vi "2-1.vi"() -> ()   [LabVIEW 2012]
doc: "© Copyright M. Ferrari 1999"
panel:
  out "Waveform Chart":dbl(graph)
  out "data out":dbl(knob) scale=0.0..10.0 scale format="%#_4g"
  out "low limit":dbl(knob) scale=10.0..100.0 scale format="%#_4g"
  out "hight limit":dbl(knob) scale=10.0..100.0 scale format="%#_4g"
  out "data in":dbl format="%.2f"
  in  "control":bool
  # "Se control = ON, bisogna verificare che il valore sia compreso nei limiti\n                     trasferendo il valore di ingresso diviso per il range ( hight limit-low limit)\n                     in uscita; se il valore  \"data in\"  non rientra nei limiti, oppure\nse control = OFF, non viene effettuato nessun controllo e il valore di ingresso passa\n                    direttamente in uscita"
  # "far apparire la scritta ON ,\no la scritta OFF, a seconda\ndei casi, su sfondo bianco"
  # "sostituire con un indicatore \ndi tipo ' meter' con indicatore digitale"
  # "sostituire con due controlli \ndi tipo ' knob' con indicatore digitale"
  # "Eliminare dal pannello tutte le indicazioni in arancio"
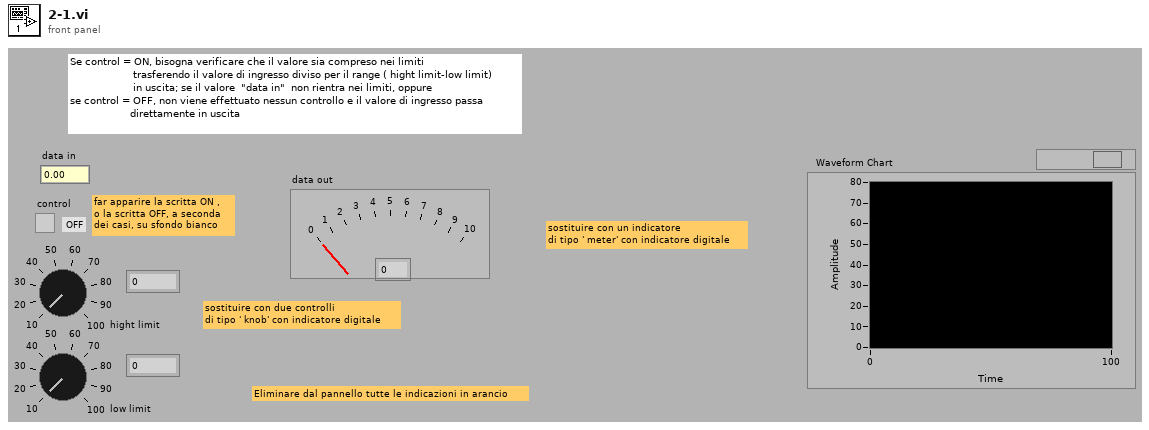
[diagram p1: front panel]
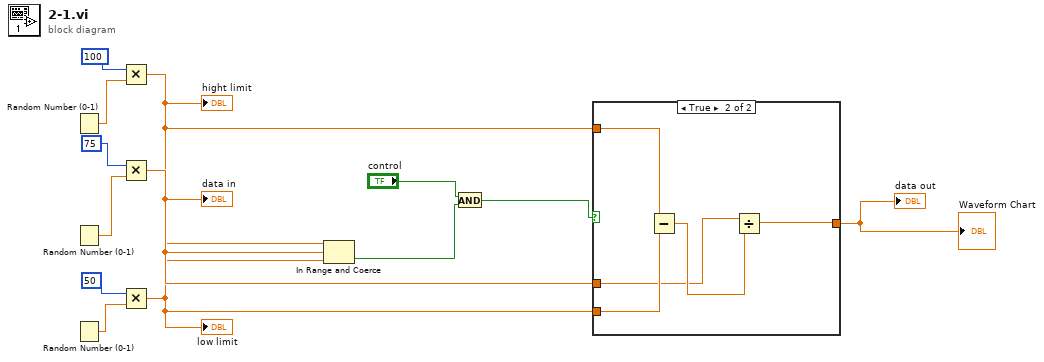
[diagram p0: block diagram]
diagram:
  n1 = Random Number (0-1)() -> (number: 0 to 1=w6:dbl)
  n2 = Random Number (0-1)() -> (number: 0 to 1=w10:dbl)
  n3 = Random Number (0-1)() -> (number: 0 to 1=w4:dbl)
  n4 = Multiply(x=100, y=w6) -> (x*y=w2:dbl)
  "hight limit" <- w2
  n5 = Multiply(x=75, y=w10) -> (x*y=w8:dbl)
  "data in" <- w8
  n6 = Multiply(x=50, y=w4) -> (x*y=w1:dbl)
  "low limit" <- w1
  n7 = In Range and Coerce(upper limit=w2, x=w8, lower limit=w1) -> (In Range?=w12:bool)  [unwired: 1 out]
  n8 = And(x="control", y=w12) -> (x .and. y?=w11:bool)
  n9 = case shown="True" w11 {
    tunnel: w8 -> [w14 w16]
    tunnel: [w14 w15] -> w7
    tunnel: w2 -> [_ w19]
    tunnel: w1 -> [_ w18]
    frame False {
    }
    frame True {
      n10 = Subtract(x=w19, y=w18) -> (x-y=w17:dbl)
      n11 = Divide(x=w16, y=w17) -> (x/y=w15:dbl)
    }
  }
  "data out" <- w7
  "Waveform Chart" <- w7
